vi "DB_Lee_Usuarios.vi"(8 "error in (no error)":errorcluster) -> (0 "error out":errorcluster, 1 "categorias":string[](array[string]), 2 "pass":string[](array[string]), 3 "usuarios":string[](array[string]))   [LabVIEW 2018]
uses:
  <vilib>/addons/database/Connection.llb/DB Tools Open Connec (Path).vi
  <vilib>/addons/database/Connection.llb/Conn Execute.vi
  <vilib>/addons/database/Recordset.llb/Rec Fetch Recordset Data (R).vi
  <vilib>/addons/database/Recordset.llb/Rec Destroy - Connection.vi
  <vilib>/addons/database/_DB Variant To Data/Database Variant To Data.xnode
  <vilib>/addons/database/NI_Database_API.lvlib
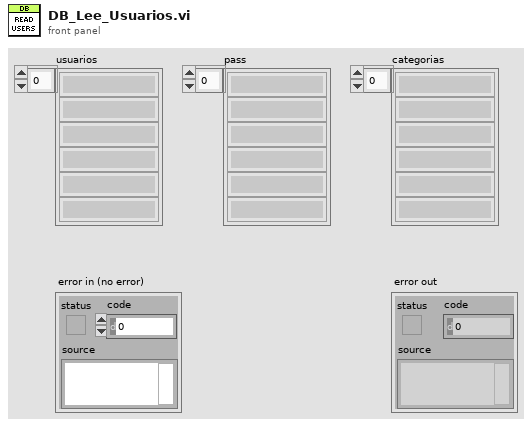
[diagram p1: front panel]
types:
  T1 = typedef "NI_Database_API.lvlib/Conn ObjectReference.ctl" = refnum<k1>
  T2 = typedef "NI_Database_API.lvlib/Rec ObjectReference.ctl" = refnum<k1>
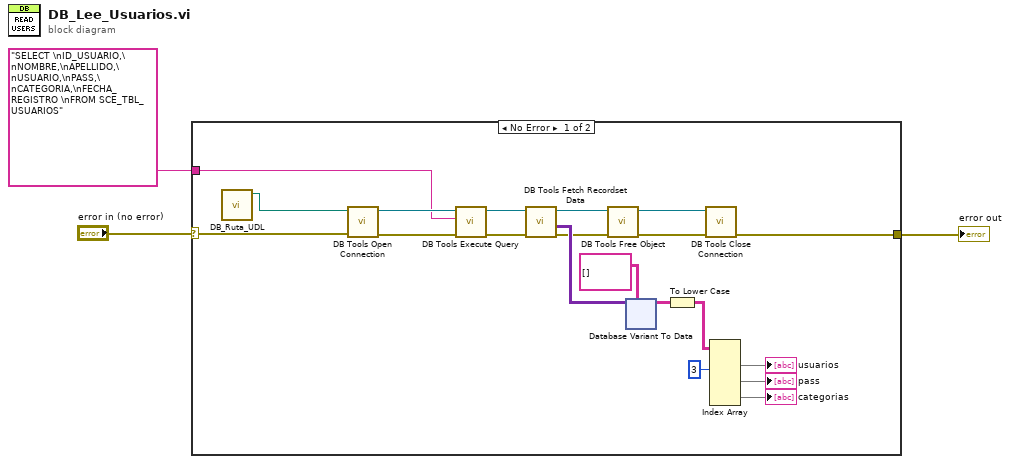
[diagram p0: block diagram]
diagram:
  n1 = case shown="No Error" "error in (no error)" {
    selector: "error in (no error)" -> [w18 w68]
    tunnel: [w20 w68] -> w3
    tunnel: "SELECT \nID_USUARIO,\nNOMBRE,\nAPELLIDO,\nUSUARIO,\nPASS,\nCATEGORIA,\nFECHA_REGISTRO \nFROM SCE_TBL_USUARIOS" ("SQL") -> [w17 _]
    frame No Error {
      n2 = call "DB_Ruta_UDL.vi"() -> ("UDL ruta"=w4:path)  [unwired: 11 in]
      n3 = call-poly <vilib>:"DB Tools Open Connection.vi"("error in (no error)"=w18, "connection information"=w4) -> ("error out"=w23:errorcluster, "connection reference"=w21:T1)  [unwired: 6 in]
      n4 = call-poly <vilib>:"DB Tools Execute Query.vi"("error in (no error)"=w23, "SQL query"=w17, "connection reference"=w21) -> ("error out"=w19:errorcluster, "recordset reference"=w16:T2)  [unwired: 5 in]
      n5 = call-poly <vilib>:"DB Tools Fetch Recordset Data.vi"("error in (no error)"=w19, "recordset reference"=w16) -> ("error out"=w12:errorcluster, "recordset data"=w13:variant[][], "recordset reference out"=w15:T2)  [unwired: 3 in]
      n6 = call-poly <vilib>:"DB Tools Free Object.vi"("error in (no error)"=w12, "recordset reference"=w15) -> ("error out"=w22:errorcluster, "connection reference"=w6:T1)  [unwired: 8 in]
      n7 = xnode "Database Variant To Data"("database variant"=w13, "type"=string[][] []) -> ("data"=w11:string[][])  [unwired: 1 in, 1 out]
      n8 = To Lower Case(string=w11) -> (all lower case string=w5:string[][])
      n9 = call <vilib>:"DB Tools Close Connection.vi"("error in (no error)"=w22, "connection reference"=w6) -> ("error out"=w20:errorcluster)  [unwired: 5 in]
      n10 = Index Array(array=w5, index (col) #1=3 ("disabled index (col)")) -> (element #1=→"usuarios":string[], element #2=→"pass":string[], element #3=→"categorias":string[])  [unwired: 5 in]
    }
    frame Error {
    }
  }
  "error out" <- w3
